vi "DualButtons.vi"() -> ()   [LabVIEW 2024]
uses:
  Driver/Public/Digital Direction.ctl
  Driver/CTIPicoVISA.lvlib
panel:
  out "Identity":T1
  in  "GroveConnector":enum16{"D16", "D18", "D20"}(ring)
  in  "stop":bool
  in  "VISA resource name in":refnum<visa-resource-name>
  out "error out":errorcluster
  out "Boolean 2":bool
  out "Boolean 1":bool
  # "https://www.seeedstudio.com/Grove-Dual-Button-p-4529.html"
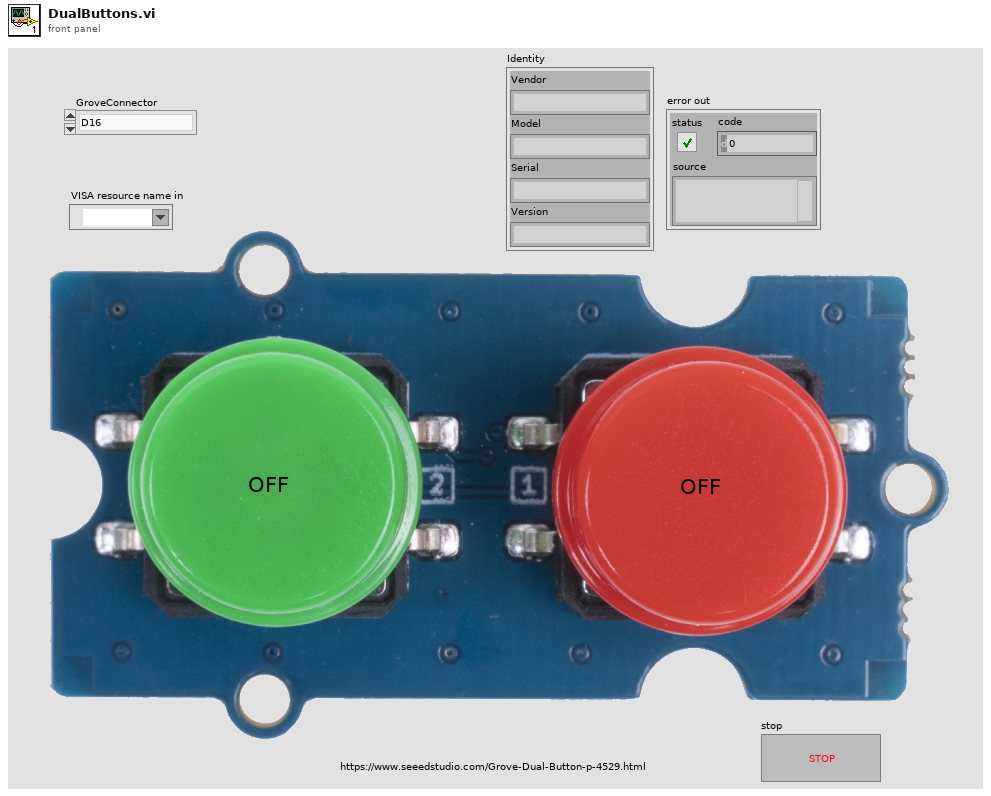
[diagram p1: front panel]
types:
  T1 = cluster{"Vendor":string, "Model":string, "Serial":string, "Version":string}
  T2 = typedef "CTIPicoVISA.lvlib/Digital Direction.ctl" = enum16{"In", "Out"}
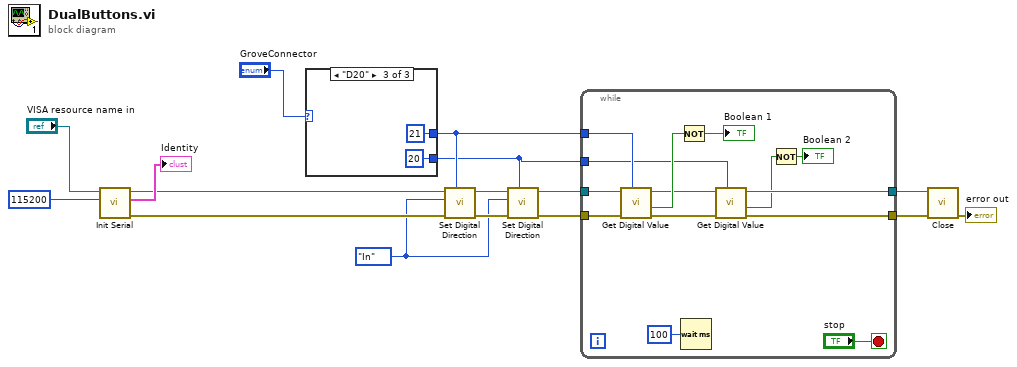
[diagram p0: block diagram]
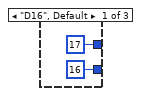
[diagram p2: hidden frame]
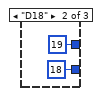
[diagram p3: hidden frame]
diagram:
  w8 = Digital_Direction."In" ("Direction")
  n1 = call "Init Serial.vi"("Baud (115200)"=u32 115200, "VISA resource name in"="VISA resource name in") -> ("error out"=w10:errorcluster, "Identity"=→"Identity":T1, "VISA resource name Out"=w12:refnum<visa-resource-name>)  [unwired: 7 in]
  n2 = case shown="\"D20\"" "GroveConnector" {
    tunnel: [17 ("GPIO") 19 ("GPIO") 21 ("GPIO")] -> w11
    tunnel: [16 ("GPIO") 18 ("GPIO") 20 ("GPIO")] -> w6
    frame "D16", Default {
    }
    frame "D18" {
    }
    frame "D20" {
    }
  }
  n3 = call "Set Digital Direction.vi"("GPIO"=w11, "error in (no error)"=w10, "Direction"=w8, "VISA resource name in"=w12) -> ("error out"=w9:errorcluster, "VISA resource name"=w7:refnum<visa-resource-name>)  [unwired: 6 in]
  n4 = call "Set Digital Direction.vi"("GPIO"=w6, "error in (no error)"=w9, "Direction"=w8, "VISA resource name in"=w7) -> ("error out"=w4:errorcluster, "VISA resource name"=w5:refnum<visa-resource-name>)  [unwired: 6 in]
  n5 = while {
    tunnel: w4 -> [w30]
    tunnel: w5 -> [w31]
    tunnel: [w25] -> w3
    tunnel: [w23] -> w2
    tunnel: w11 -> [w32]
    tunnel: w6 -> [w26]
    stop <- "stop" stop-if-true
    n6 = call "Get Digital Value.vi"("GPIO"=w32, "error in (no error)"=w30, "VISA resource name in"=w31) -> ("error out"=w27:errorcluster, "Value"=w29:bool, "VISA resource name"=w28:refnum<visa-resource-name>)  [unwired: 6 in]
    n7 = Not(x=w29) -> (.not. x?=→"Boolean 1":bool)
    n8 = Wait (ms)(milliseconds to wait=u32 100) -> ()  [unwired: 1 out]
    n9 = call "Get Digital Value.vi"("GPIO"=w26, "error in (no error)"=w27, "VISA resource name in"=w28) -> ("error out"=w23:errorcluster, "Value"=w24:bool, "VISA resource name"=w25:refnum<visa-resource-name>)  [unwired: 6 in]
    n10 = Not(x=w24) -> (.not. x?=→"Boolean 2":bool)
  }
  n11 = call "Close.vi"("error in (no error)"=w2, "VISA resource name in"=w3) -> ("error out"=→"error out":errorcluster)  [unwired: 9 in]
